vi "MCT FTP Upload.vi"(7 "슬라이드":refnum<vi>, 8 "error in":errorcluster caption="에러 입력(에러 없음)") -> (0 "error out":errorcluster caption="에러 출력", 3 "이후 Version":string)   [LabVIEW 2020]
uses:
  Controls/Cmd_File path.ctl
  Controls/Cmd_File Type.ctl
  Controls/Cmd_Write Query.ctl
  Controls/Clst_Query Info.ctl
  <vilib>/Utility/error.llb/Error Cluster From Error Code.vi
  Public/Polymorph/ini Ctrl_Str.vi
  <vilib>/ErrorRing/Error Ring.xnode
  <vilib>/addons/database/NI_Database_API.lvlib
  <vilib>/FTP/NI_FTP.lvlib
panel:
  out "이전 Version":string
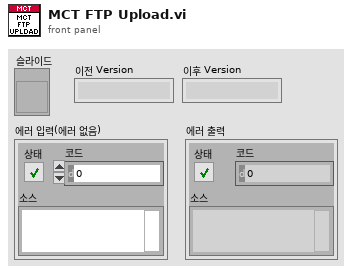
[diagram p1: front panel]
types:
  T1 = typedef "Cmd_File path.ctl" = enum16{"에러로그", "데이터파일경로", "성적서원본", "지난성적서", "Data Files", "경로생성", "Updater", "Template", "설정파일경로", "FTP Upload", "Update 경로", "어플리케이션"}
  T2 = typedef "NI_FTP.lvlib/FTP Session.ctl" = refnum<k5>
  T3 = cluster{"로컬경로":path, "원격경로":string, "MD5 message-digest":string}
  T4 = typedef "Cmd_File Type.ctl" = enum16{"엑셀", "엑셀(2003)", "텍스트", "설정", "2진", "VI", "CSV", "LOG", "폴더"}
  T5 = enum16{"open", "replace", "create", "open or create", "replace or create", "replace or create with confirmation"}
  T6 = typedef "Clst_Query Info.ctl" = cluster{"사번":string, "등록번호":string, "업체명":string, "세부분류코드":string, "형식":string, "기기번호":string, "FUNC":string, "FUNC_EXT":string, "옵션":string, "추가문자열":string, "일자":string, "배열 1":string[], "배열 2":string[], "항목명":string, "문자열":string, "이름":string}
  T7 = typedef "Cmd_Write Query.ctl" = enum16{"TBUSESTD_MCT Insert", "TBUSESTD_MCT Delete", "TBCALSTD_MCT_TEMP Insert", "TBCALSTD_MCT_TEMP Delete", "TBCALSTD_MCT Insert", "TBCALSTD_MCT Delete", "TBCALSTD_MCT_BACK Insert", "TBCALSTD_MCT_BACK Delete", "TBCALPROC_MCT Insert", "TBCALPROC_MCT Delete", "TBCALPROC_MCT_TEMP Insert", "TBCALPROC_MCT_TEMP Delete", "TBCALCMC_MCT Insert", "TBCALCMC_MCT Delete", "TBCALFUNC_MCT Insert", "TBCALFUNC_MCT Delete", "TBCALNAME_MCT Insert", "TBCALNAME_MCT Delete", "TBSTDNAME_MCT Insert", "TBSTDNAME_MCT Delete", "TBCALSPEC_MCT Insert", "TBCALSPEC_MCT Delete", "TBCALSTD_MCT NOTUSE update", "TBCALSPEC_MCT update", "TBMCTVERMAN update"}
  T8 = typedef "NI_Database_API.lvlib/Conn ObjectReference.ctl" = refnum<k1>
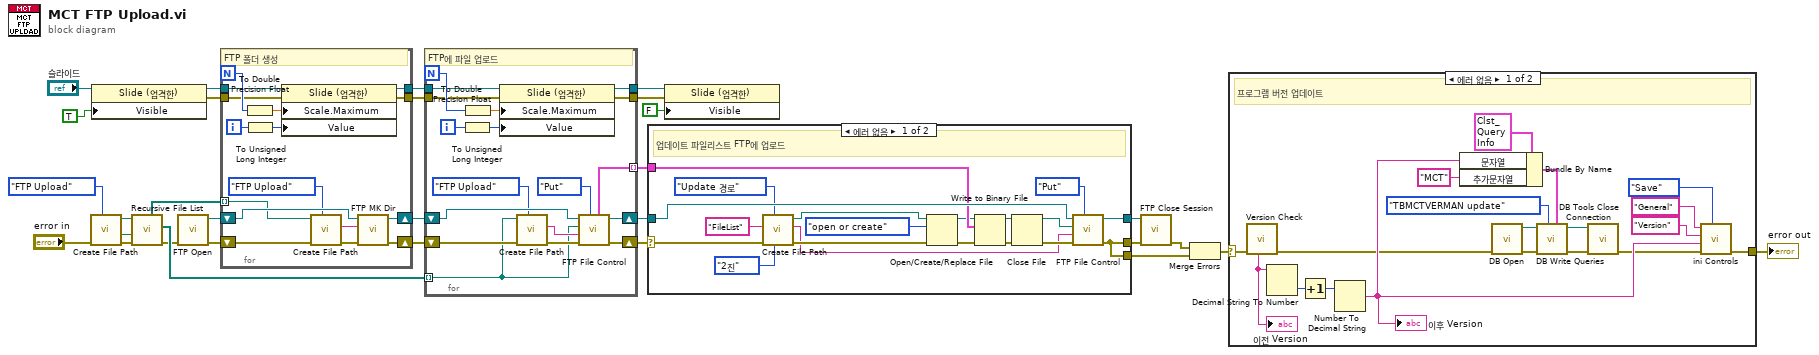
[diagram p0: block diagram]
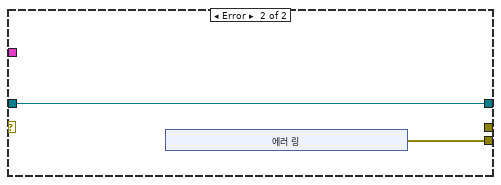
[diagram p3: hidden frame]
diagram:
  n1 = call "Create File Path.vi"("항목"=Cmd_File_path."FTP Upload", "에러 입력"="error in") -> ("error out"=w9:errorcluster, "파일존재?"=w12:bool, "파일경로"=w8:path)  [unwired: 6 in, 1 out]
  n2 = property class="Slide (엄격한)"(reference="슬라이드", "Visible"=TRUE ("보이기")) -> (reference out=w18:refnum<vi>, error out=w19:errorcluster)  [unwired: 1 in]
  n3 = call <vilib>:"Recursive File List.vi"("error in (no error)"=w9, "Continue Recursing on Error? (F)"=w12, "Folder Path"=w8) -> ("error out"=w20:errorcluster, "All Files in Dir"=w29:path[], "All Folders"=w30:path[])  [unwired: 4 in, 2 out]
  n4 = call "FTP Open.vi"("에러 입력(에러 없음)"=w20) -> ("에러 출력"=w6:errorcluster, "TCP 네트워크 연결 출력"=w7:T2)  [unwired: 9 in]
  n5 = for {
    N -> [w43]
    tunnel: w30 -> [w32] mode=indexing
    shift-right: [w46] -> w28
    shift-left: w6 -> [w34]
    shift-right: [w44] -> w27
    shift-left: w7 -> [w45]
    tunnel: w19 -> [w39]
    tunnel: w18 -> [w38]
    tunnel: [w37] -> w16
    tunnel: [w36] -> w17
    i -> [w41]
    # "FTP 폴더 생성"
    n6 = To Double Precision Float(number=w43) -> (double precision float=w42:dbl)
    n7 = To Unsigned Long Integer(number=w41) -> (unsigned 32bit integer=w40:u32)
    n8 = property class="Slide (엄격한)"(reference=w38, error in=w39, "Scale.Maximum"=w42, "Value"=w40) -> (reference out=w36:refnum<vi>, error out=w37:errorcluster)
    n9 = call "Create File Path.vi"("항목"=Cmd_File_path."FTP Upload", "에러 입력"=w34, "폴더명 in"=w32) -> ("error out"=w33:errorcluster, "문자열 out"=w31:string)  [unwired: 5 in, 2 out]
    n10 = call "FTP MK Dir.vi"("에러 입력(에러 없음)"=w33, "디렉토리명"=w31, "ftp session"=w45) -> ("에러 출력"=w46:errorcluster, "ftp session out"=w44:T2)  [unwired: 7 in]
  }
  n11 = for {
    N -> [w58]
    shift-right: [w49] -> w15
    shift-left: w28 -> [w51]
    tunnel: w29 -> [w47] mode=indexing
    shift-right: [w62] -> w25
    shift-left: w27 -> [w63]
    tunnel: [w61] -> w24 mode=indexing
    tunnel: w17 -> [w56]
    tunnel: w16 -> [w55]
    tunnel: [w54] -> w13
    tunnel: [w53] -> w14
    i -> [w60]
    # "FTP에 파일 업로드"
    n12 = To Unsigned Long Integer(number=w60) -> (unsigned 32bit integer=w59:u32)
    n13 = To Double Precision Float(number=w58) -> (double precision float=w57:dbl)
    n14 = property class="Slide (엄격한)"(reference=w56, error in=w55, "Scale.Maximum"=w57, "Value"=w59) -> (reference out=w54:refnum<vi>, error out=w53:errorcluster)
    n15 = call "Create File Path.vi"("항목"=Cmd_File_path."FTP Upload", "에러 입력"=w51, "폴더명 in"=w47) -> ("문자열 out"=w48:string)  [unwired: 5 in, 3 out]
    n16 = call "FTP File Control.vi"("Comm"=enum16{"Get", "Put"}."Put", "에러 입력"=w51, "원격경로"=w48, "로컬경로"=w47, "TCP 네트워크 연결 입력"=w63) -> ("에러 출력"=w49:errorcluster, "TCP 네트워크 연결 출력"=w62:T2, "출력 클러스터"=w61:T3)  [unwired: 2 in, 2 out]
  }
  n17 = case shown="에러 없음" w15 {
    selector: w15 -> [w71 _]
    tunnel: w25 -> [w82 w83]
    tunnel: w24 -> [w81 _]
    tunnel: [w64 w84] -> w2
    tunnel: [w65 w83] -> w5
    tunnel: [w64 _] -> w1
    frame No Error {
      # "업데이트 파일리스트 FTP에 업로드"
      n18 = call "Create File Path.vi"("파일타입"=Cmd_File_Type."2진", "항목"=Cmd_File_path."Update 경로", "에러 입력"=w71, "문자열 in"="FileList" ("이름 또는 상대 경로")) -> ("error out"=w75:errorcluster, "문자열 out"=w66:string, "파일경로"=w70:path)  [unwired: 4 in, 1 out]
      n19 = Open/Create/Replace File(file path (use dialog)=w70, error in=w75, operation (0:open)=T5."open or create" ("동작(0:open)")) -> (refnum out=w78:refnum<file>, error out=w77:errorcluster)  [unwired: 3 in, 1 out]
      n20 = Write to Binary File(file (use dialog)=w78, data=w81, error in=w77) -> (refnum out=w79:refnum<file>, error out=w80:errorcluster)  [unwired: 3 in, 1 out]
      n21 = Close File(refnum=w79, error in=w80) -> (path=w67:path, error out=w74:errorcluster)
      n22 = call "FTP File Control.vi"("Comm"=enum16{"Get", "Put"}."Put", "에러 입력"=w74, "원격경로"=w66, "로컬경로"=w67, "TCP 네트워크 연결 입력"=w82) -> ("에러 출력"=w64:errorcluster, "TCP 네트워크 연결 출력"=w65:T2)  [unwired: 2 in, 3 out]
    }
    frame Error {
      n23 = xnode "에러 링"() -> ("에러 출력"=w84:errorcluster)
    }
  }
  n24 = property class="Slide (엄격한)"(reference=w13, error in=w14, "Visible"=FALSE ("보이기")) -> ()  [unwired: 2 out]
  n25 = call <vilib>:"FTP Close Session.vi"("error in (no error)"=w1, "ftp session"=w5) -> ("error out"=w4:errorcluster)  [unwired: 6 in, 3 out]
  n26 = Merge Errors(w4, w2) -> (w3:errorcluster)
  n27 = case shown="에러 없음" w3 {
    selector: w3 -> [w106 w109]
    tunnel: [w108 w109] -> w26
    frame No Error {
      # "프로그램 버전 업데이트"
      n28 = call "Version Check.vi"("에러 입력"=w106) -> ("에러 출력"=w95:errorcluster, "MCT 서버버전"=w105:string)  [unwired: 4 in, 5 out]
      "이전 Version" <- w105
      n29 = Decimal String To Number(string=w105) -> (number=w104:i32)  [unwired: 2 in, 1 out]
      n30 = Increment(x=w104) -> (x+1=w103:i32)
      n31 = Number To Decimal String(number=w103) -> (decimal integer string=w107:string)  [unwired: 1 in]
      "이후 Version" <- w107
      n32 = Bundle By Name(cluster=T6 {"사번"="", "등록번호"="", "업체명"="", "세부분류코드"="", "형식"="", "기기번호"="", "FUNC"="", "FUNC_EXT"="", "옵션"="", "추가문자열"="", "일자"="", "배열 1"=[], "배열 2"=[], "항목명"="", "문자열"="", "이름"=""} ("Query info"), "문자열"=w107, "추가문자열"="MCT") -> (w96:T6)
      n33 = call "DB Open.vi"("에러 입력"=w95) -> ("에러 출력"=w101:errorcluster, "참조 번호 출력"=w102:T8)  [unwired: 9 in]
      n34 = call "DB Write Queries.vi"("Query info"=w96, "COMMAND"=Cmd_Write_Query."TBMCTVERMAN update", "에러 입력(에러 없음)"=w101, "참조 번호 입력"=w102) -> ("에러 출력"=w99:errorcluster, "참조 번호 출력"=w100:T8)  [unwired: 6 in]
      n35 = call <vilib>:"DB Tools Close Connection.vi"("error in (no error)"=w99, "connection reference"=w100) -> ("error out"=w90:errorcluster)  [unwired: 5 in]
      n36 = call-poly "ini Controls.vi"("Select"=enum16{"Save", "Load"}."Save", "에러 입력"=w90, "값"=w107, "키"="Version" ("key"), "섹션"="General" ("section")) -> ("에러 출력"=w108:errorcluster)  [unwired: 4 in, 2 out]
    }
    frame Error {
    }
  }
  "error out" <- w26
